vi "YAG_Control.v3.vi"() -> ()   [LabVIEW 2018]
panel:
  in  "VISA resource name":refnum<visa-resource-name>="COM1"
  in  "Cluster":T1={"Lamp mode"=TRUE, "Lamps"=FALSE, "Shutter"=FALSE, "Q-Switch"=FALSE, "Int Rep Rate  "=15.0, "Voltage "=700.0, "Temperature"=20.0, "Quit"=FALSE} {"Int Rep Rate" min=1.0 max=30.0; "Temperature" format="%#.0f"; "Voltage" min=680.0 max=1100.0}
  in  "Send":bool
  out "Last Response":string
  in  "Other Command":string
  # "o"
  # "C"
  # "Hz"
  # "V"
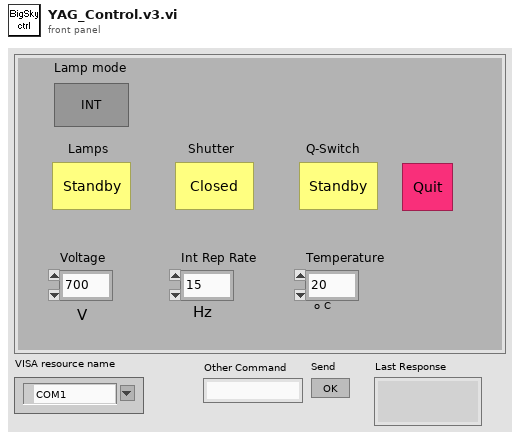
[diagram p1: front panel]
types:
  T1 = cluster{"Lamp mode":bool, "Lamps":bool, "Shutter":bool, "Q-Switch":bool, "Int Rep Rate  ":dbl, "Voltage ":dbl, "Temperature":dbl, "Quit":bool}
  T2 = enum8{"Enabled", "Disabled", "Disabled and Grayed Out"}
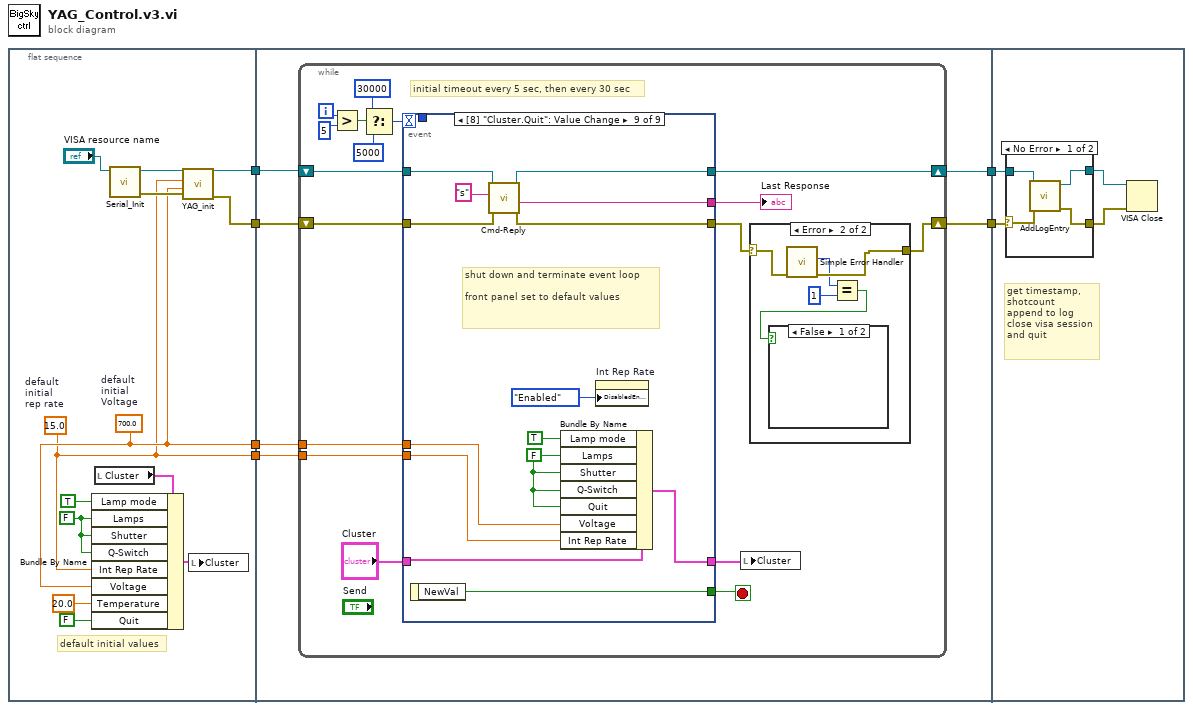
[diagram p0: block diagram]
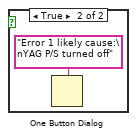
[diagram p3: hidden frame]
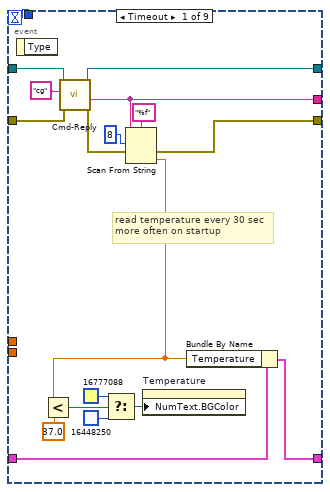
[diagram p4: hidden frame]
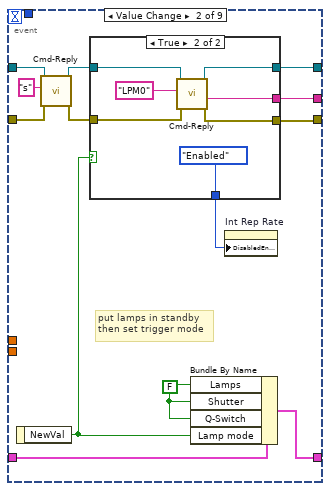
[diagram p5: hidden frame]
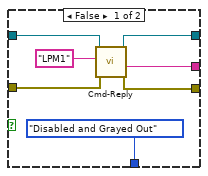
[diagram p6: hidden frame]
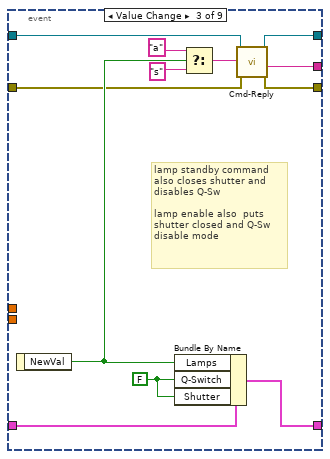
[diagram p7: hidden frame]
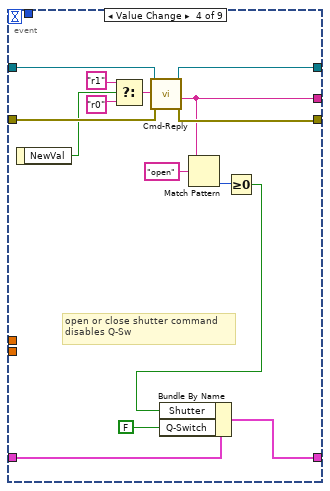
[diagram p8: hidden frame]
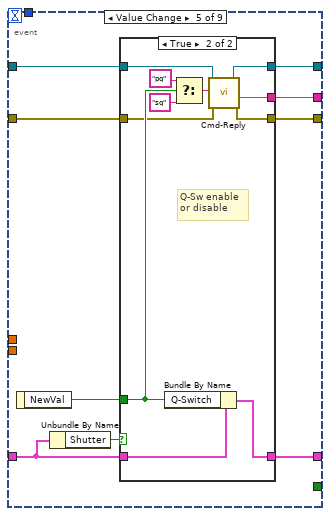
[diagram p9: hidden frame]
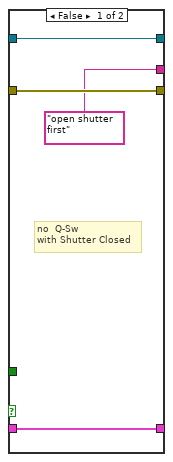
[diagram p10: hidden frame]
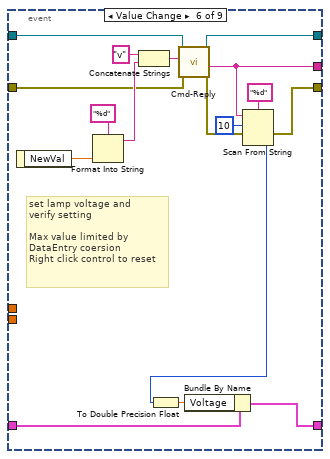
[diagram p11: hidden frame]
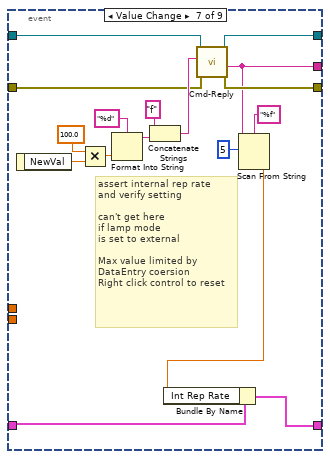
[diagram p12: hidden frame]
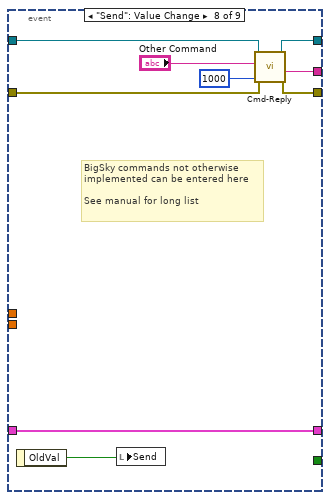
[diagram p13: hidden frame]
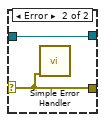
[diagram p14: hidden frame]
diagram:
  n1 = flat-sequence {
    tunnel: [w17] -> w4
    tunnel: [w10] -> w3
    tunnel: [w8] -> w2
    tunnel: [w7] -> w1
    tunnel: [w25] -> w6
    tunnel: [w24] -> w5
    tunnel: w4 -> [w23]
    tunnel: w3 -> [w22]
    tunnel: w2 -> [w21]
    tunnel: w1 -> [w20]
    tunnel: w6 -> [w203]
    tunnel: w5 -> [w206]
    frame #0 {
      w7 = 15.0  # default initial rep rate
      w8 = 700.0  # default  initial Voltage
      w14 = FALSE ("Lamp mode")
      # "default initial values"
      n2 = local read "Cluster"() -> (w15:T1)
      n3 = Bundle By Name(cluster=w15, "Lamp mode"=TRUE, "Lamps"=w14, "Shutter"=w14, "Q-Switch"=w14, "Int Rep Rate"=w7, "Voltage"=w8, "Temperature"=20.0, "Quit"=FALSE) -> (w11:T1)
      n4 = call "Serial_Init.vi"("VISA resource name"="VISA resource name") -> ("error out"=w16:errorcluster, "VISA resource name out"=w18:refnum<visa-resource-name>)  [unwired: 9 in]
      n5 = call "YAG_init.vi"("error in (no error)"=w16, "initial V"=w8, "initial rep rate"=w7, "VISA Refnum in"=w18) -> ("error out"=w10:errorcluster, "VISA Refnum out"=w17:refnum<visa-resource-name>)  [unwired: 6 in]
      n6 = local write "Cluster"(w11) -> ()
    }
    frame #1 {
      n7 = while {
        shift-right: [w36] -> w24
        shift-left: w23 -> [w38]
        shift-right: [w34] -> w25
        shift-left: w22 -> [w37]
        tunnel: w21 -> [w27]
        tunnel: w20 -> [w26]
        i -> [w30]
        stop <- w42 stop-if-true
        # "initial timeout every 5 sec, then every 30 sec"
        n8 = Greater?(x=w30, y=5) -> (0:w28:bool)
        n9 = Select(t=30000, s=w28, f=5000) -> (s? t:f=w33:i32)
        n10 = event shown="[8] \"Cluster.Quit\": Value Change" {
          selector: _ -> [_ _ _ _ _ _ _ _ _]
          dyn-events: _ -> [_ _ _ _ _ _ _ _ _]
          timeout: w33 -> [w51 _ _ _ _ _ _ _ _]
          tunnel: [_ _ _ _ _ _ _ _ w200] -> w42
          tunnel: "Cluster" -> [w67 w80 w106 w121 w128 w146 w178 w188 w202]
          tunnel: [w66 w79 w101 w120 w130 w162 w177 w188 w201] -> w39
          tunnel: [w61 w77 w100 w111 w126 w152 w167 w186 w194] -> w41
          tunnel: w38 -> [w63 w72 w96 w114 w122 w154 w169 w184 w197]
          tunnel: w37 -> [w64 w69 w97 w113 w123 w156 w168 w183 w198]
          tunnel: [w58 w73 w98 w115 w124 w148 w176 w182 w193] -> w35
          tunnel: [w62 w74 w99 w116 w125 w155 w175 w181 w195] -> w36
          tunnel: [w51 _ _ _ _ _ _ _ _] -> _
          tunnel: w27 -> [_ _ _ _ _ _ _ _ w190]
          tunnel: w26 -> [_ _ _ _ _ _ _ _ w189]
          event Timeout {
            # "read temperature every 30 sec\nmore often on startup"
            n11 = event-data() -> ()  [unwired: 1 in, 1 out]
            n12 = call "Cmd-Reply.vi"("error in (no error)"=w64, "cmd"="cg" ("write buffer"), "VISA Refnum in"=w63) -> ("error out"=w59:errorcluster, "reply"=w61:string, "VISA Refnum out"=w62:refnum<visa-resource-name>)  [unwired: 6 in]
            n13 = Scan From String(format string="%f", input string=w61, initial scan location=u32 8, error in=w59) -> (error out=w58:errorcluster, output 1=w57:dbl)  [unwired: 1 in, 2 out]
            n14 = Less?(x=w57, y=37.0) -> (x < y?=w54:bool)
            n15 = Select(t=u32 16777088 ("Color"), s=w54, f=u32 16448250 ("Color")) -> (s? t:f=w55:u32)
            n16 = property on="Temperature" class="DigNum (strict)"("NumText.BGColor"=w55) -> ()  [unwired: 2 in, 2 out]
            n17 = Bundle By Name(cluster=w67, "Temperature"=w57) -> (w66:T1)
          }
          event "Cluster.Lamp mode": Value Change {
            w78 = FALSE
            # "put lamps in standby\nthen set trigger mode"
            n18 = event-data() -> ("NewVal"=w75:bool)  [unwired: 1 in]
            n19 = call "Cmd-Reply.vi"("error in (no error)"=w69, "cmd"="s" ("write buffer"), "VISA Refnum in"=w72) -> ("error out"=w68:errorcluster, "VISA Refnum out"=w71:refnum<visa-resource-name>)  [unwired: 6 in, 1 out]
            n20 = case shown="True" w75 {
              tunnel: [w86 w88] -> w77
              tunnel: [T2."Disabled and Grayed Out" ("Disabled") T2."Enabled" ("Disabled")] -> w76
              tunnel: [w85 w91] -> w74
              tunnel: [w84 w89] -> w73
              tunnel: w71 -> [w83 w92]
              tunnel: w68 -> [w82 w90]
              frame False {
                n21 = call "Cmd-Reply.vi"("error in (no error)"=w82, "cmd"="LPM1", "VISA Refnum in"=w83) -> ("error out"=w84:errorcluster, "reply"=w86:string, "VISA Refnum out"=w85:refnum<visa-resource-name>)  [unwired: 6 in]
              }
              frame True {
                n22 = call "Cmd-Reply.vi"("error in (no error)"=w90, "cmd"="LPM0", "VISA Refnum in"=w92) -> ("error out"=w89:errorcluster, "reply"=w88:string, "VISA Refnum out"=w91:refnum<visa-resource-name>)  [unwired: 6 in]
              }
            }
            n23 = Bundle By Name(cluster=w80, "Lamps"=w78, "Shutter"=w78, "Q-Switch"=w78, "Lamp mode"=w75) -> (w79:T1)
            n24 = property on="Int Rep Rate" class="DigNum (strict)"("DisabledEnum"=w76) -> ()  [unwired: 2 in, 2 out]
          }
          event "Cluster.Lamps": Value Change {
            w102 = FALSE
            # "lamp standby command\nalso closes shutter and\ndisables Q-Sw\n\nlamp enable also  puts\nshutter closed and Q-Sw \ndisable mode"
            n25 = event-data() -> ("NewVal"=w103:bool)  [unwired: 1 in]
            n26 = Bundle By Name(cluster=w106, "Lamps"=w103, "Q-Switch"=w102, "Shutter"=w102) -> (w101:T1)
            n27 = Select(t="a", s=w103, f="s") -> (s? t:f=w95:string)
            n28 = call "Cmd-Reply.vi"("error in (no error)"=w97, "cmd"=w95, "VISA Refnum in"=w96) -> ("error out"=w98:errorcluster, "reply"=w100:string, "VISA Refnum out"=w99:refnum<visa-resource-name>)  [unwired: 6 in]
          }
          event "Cluster.Shutter": Value Change {
            # "open or close shutter command\ndisables Q-Sw"
            n29 = event-data() -> ("NewVal"=w108:bool)  [unwired: 1 in]
            n30 = Select(t="r1", s=w108, f="r0") -> (s? t:f=w112:string)
            n31 = call "Cmd-Reply.vi"("error in (no error)"=w113, "cmd"=w112, "VISA Refnum in"=w114) -> ("error out"=w115:errorcluster, "reply"=w111:string, "VISA Refnum out"=w116:refnum<visa-resource-name>)  [unwired: 6 in]
            n32 = Match Pattern(string=w111, regular expression="open") -> (offset past match=w109:i32)  [unwired: 1 in, 3 out]
            n33 = Greater Or Equal To 0?(x=w109) -> (x >= 0?=w107:bool)
            n34 = Bundle By Name(cluster=w121, "Shutter"=w107, "Q-Switch"=FALSE) -> (w120:T1)
          }
          event "Cluster.Q-Switch": Value Change {
            n35 = event-data() -> ("NewVal"=w129:bool)  [unwired: 1 in]
            n36 = Unbundle By Name(w128) -> ("Shutter"=w127:bool)
            n37 = case shown="True" w127 {
              tunnel: [w134 w141] -> w130
              tunnel: w129 -> [_ w142]
              tunnel: w128 -> [w134 w145]
              tunnel: ["open shutter first" w140] -> w126
              tunnel: [w133 w139] -> w125
              tunnel: [w132 w138] -> w124
              tunnel: w123 -> [w132 w137]
              tunnel: w122 -> [w133 w136]
              frame False {
                # "no  Q-Sw \nwith Shutter Closed"
              }
              frame True {
                # "Q-Sw enable\nor disable"
                n38 = Bundle By Name(cluster=w145, "Q-Switch"=w142) -> (w141:T1)
                n39 = Select(t="pq", s=w142, f="sq") -> (s? t:f=w135:string)
                n40 = call "Cmd-Reply.vi"("error in (no error)"=w137, "cmd"=w135, "VISA Refnum in"=w136) -> ("error out"=w138:errorcluster, "reply"=w140:string, "VISA Refnum out"=w139:refnum<visa-resource-name>)  [unwired: 6 in]
              }
            }
          }
          event "Cluster.Voltage": Value Change {
            # "set lamp voltage and\nverify setting\n\nMax value limited by\nDataEntry coersion \nRight click control to reset"
            n41 = event-data() -> ("NewVal"=w160:dbl)  [unwired: 1 in]
            n42 = Format Into String(format string="%d", w160) -> (resulting string=w158:string)  [unwired: 2 in, 1 out]
            n43 = Concatenate Strings("v" ("string"), w158) -> (w159:string)
            n44 = call "Cmd-Reply.vi"("error in (no error)"=w156, "cmd"=w159, "VISA Refnum in"=w154) -> ("error out"=w149:errorcluster, "reply"=w152:string, "VISA Refnum out"=w155:refnum<visa-resource-name>)  [unwired: 6 in]
            n45 = Scan From String(format string="%d", input string=w152, initial scan location=u32 10, error in=w149) -> (error out=w148:errorcluster, output 1=w153:i32)  [unwired: 1 in, 2 out]
            n46 = To Double Precision Float(number=w153) -> (double precision float=w147:dbl)
            n47 = Bundle By Name(cluster=w146, "Voltage"=w147) -> (w162:T1)
          }
          event "Cluster.Int Rep Rate": Value Change {
            # "assert internal rep rate\nand verify setting\n\ncan't get here  \nif lamp mode\nis set to external\n\nMax value limited by\nDataEntry coersion \nRight click control to reset"
            n48 = event-data() -> ("NewVal"=w164:dbl)  [unwired: 1 in]
            n49 = Multiply(x=100.0, y=w164) -> (x*y=w172:dbl)
            n50 = Format Into String(format string="%d", w172) -> (resulting string=w170:string)  [unwired: 2 in, 1 out]
            n51 = Concatenate Strings("f" ("string"), w170) -> (w174:string)
            n52 = call "Cmd-Reply.vi"("error in (no error)"=w168, "cmd"=w174, "VISA Refnum in"=w169) -> ("error out"=w176:errorcluster, "reply"=w167:string, "VISA Refnum out"=w175:refnum<visa-resource-name>)  [unwired: 6 in]
            n53 = Scan From String(format string="%f", input string=w167, initial scan location=u32 5) -> (output 1=w163:dbl)  [unwired: 2 in, 3 out]
            n54 = Bundle By Name(cluster=w178, "Int Rep Rate"=w163) -> (w177:T1)
          }
          event "Send": Value Change {
            # "BigSky commands not otherwise\nimplemented can be entered here\n\nSee manual for long list"
            n55 = event-data() -> ("OldVal"=w187:bool)  [unwired: 1 in]
            n56 = local write "Send"(w187) -> ()
            n57 = call "Cmd-Reply.vi"("error in (no error)"=w183, "ms to wait"=u32 1000, "cmd"="Other Command", "VISA Refnum in"=w184) -> ("error out"=w182:errorcluster, "reply"=w186:string, "VISA Refnum out"=w181:refnum<visa-resource-name>)  [unwired: 5 in]
          }
          event "Cluster.Quit": Value Change {
            w199 = FALSE
            # "shut down and terminate event loop\n\nfront panel set to default values"
            n58 = event-data() -> ("NewVal"=w200:bool)  [unwired: 1 in]
            n59 = call "Cmd-Reply.vi"("error in (no error)"=w198, "cmd"="s", "VISA Refnum in"=w197) -> ("error out"=w193:errorcluster, "reply"=w194:string, "VISA Refnum out"=w195:refnum<visa-resource-name>)  [unwired: 6 in]
            n60 = Bundle By Name(cluster=w202, "Lamp mode"=TRUE, "Lamps"=w199, "Shutter"=w199, "Q-Switch"=w199, "Quit"=w199, "Voltage"=w190, "Int Rep Rate"=w189) -> (w201:T1)
            n61 = property on="Int Rep Rate" class="DigNum (strict)"("DisabledEnum"=T2."Enabled" ("Disabled")) -> ()  [unwired: 2 in, 2 out]
          }
        }
        "Last Response" <- w41
        n62 = local write "Cluster"(w39) -> ()
        n63 = case shown="Error" w35 {
          selector: w35 -> [w43 w48]
          tunnel: [w43 w47] -> w34
          frame No Error {
          }
          frame Error {
            n64 = call <vilib>:"Simple Error Handler.vi"("error in (no error)"=w48) -> ("code out"=w46:i32, "error out"=w47:errorcluster)  [unwired: 4 in, 3 out]
            n65 = Equal?(x=w46, y=1) -> (x = y?=w44:bool)
            n66 = case shown="False" w44 {
              frame False {
              }
              frame True {
                n67 = One Button Dialog(message="Error 1 likely cause:\nYAG P/S turned off") -> ()  [unwired: 1 in, 1 out]
              }
            }
          }
        }
      }
    }
    frame #2 {
      # "get timestamp,\nshotcount\nappend to log\nclose visa session\nand quit"
      n68 = case shown="No Error" w203 {
        selector: w203 -> [w207 w211]
        tunnel: w206 -> [w210 w212]
        tunnel: [w209 w211] -> w205
        tunnel: [w208 w212] -> w204
        frame No Error {
          n69 = call "AddLogEntry.vi"("error in"=w207, "VISA Refnum in"=w210) -> ("error out"=w209:errorcluster, "VISA Refnum out"=w208:refnum<visa-resource-name>)  [unwired: 8 in]
        }
        frame Error {
          n70 = call <vilib>:"Simple Error Handler.vi"("error in (no error)"=w211) -> ()  [unwired: 4 in, 5 out]
        }
      }
      n71 = VISA Close(VISA resource name=w204, error in (no error)=w205) -> ()  [unwired: 1 out]
    }
  }
